vi "ExampleGreyscaleImageData.vi"(8 "error in (no error)":errorcluster, 11 "Image Size":T3={"Width"=3, "Height"=2}) -> (0 "error out":errorcluster, 3 "Greyscale Destination Image":T1, 5 "Greyscale Data":u8[][](array[numeric]), 7 "Greyscale Pixmap Data":T2)   [LabVIEW 2020, in "test.lvlib" / "01_Image.lvclass"]
uses:
  01_Image.lvclass
  common/Image Size (Integer).ctl
  <vilib>/picture/picture.llb/imagedata.ctl
  image/Greyscale Image.ctl
  image/New Image (Greyscale Preallocated).vi
  image/Copy Array to Image (Greyscale).vi
  image/New Image (Greyscale Preallocated).vi/6598b9e0-8a08-46f5-91fd-ca1b87217137.vi
  <vilib>/Utility/error.llb/Error Cluster From Error Code.vi
  01_Image.lvclass/01_Image.ctl
  image/image.lvlib
  common/common.lvlib
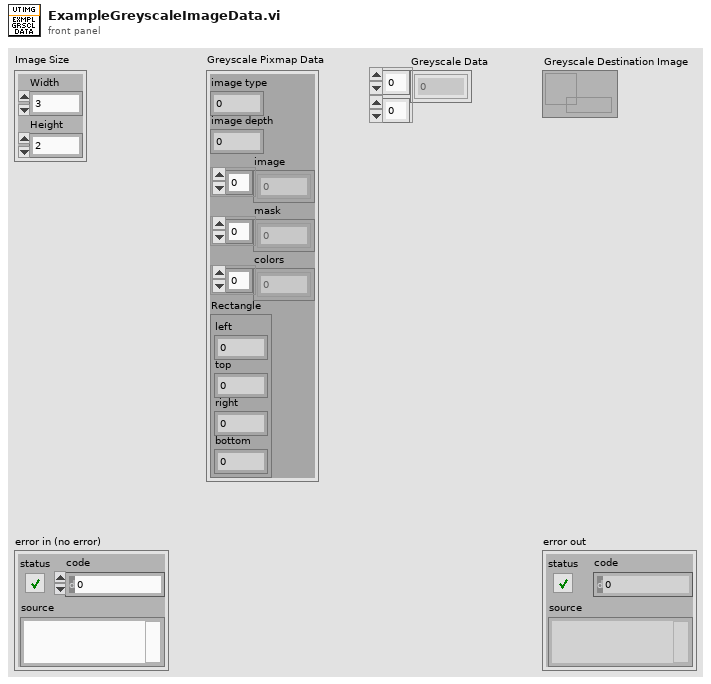
[diagram p1: front panel]
types:
  T1 = typedef "image.lvlib/Greyscale Image.ctl" = refnum<data-value>
  T2 = typedef "imagedata.ctl" = cluster{"image type":i32, "image depth":i32, "image":u8[], "mask":u8[], "colors":u32[], "Rectangle":cluster{"left":i16, "top":i16, "right":i16, "bottom":i16}}
  T3 = typedef "common.lvlib/Image Size (Integer).ctl" = cluster{"Width":u16, "Height":u16}
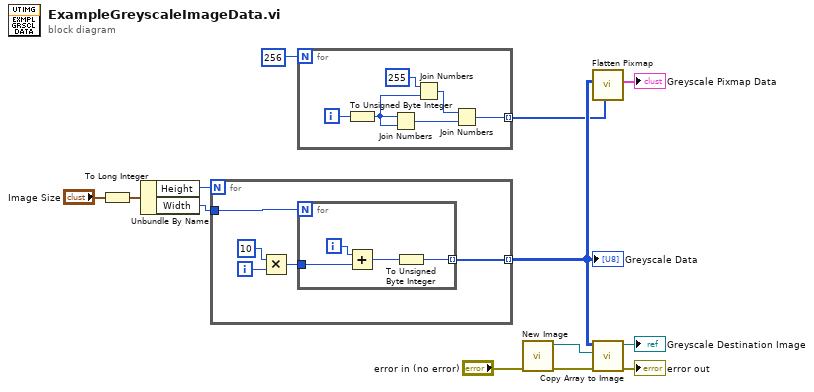
[diagram p0: block diagram]
diagram:
  n1 = To Long Integer(number="Image Size") -> (32bit integer=w12:cluster{"Width":i32, "Height":i32})
  n2 = Unbundle By Name(w12) -> ("Height"=w6:i32, "Width"=w5:i32)
  n3 = for {
    N: w6 -> [_]
    tunnel: w5 -> [w18]
    tunnel: [w14] -> w4 mode=indexing
    i -> [w17]
    n4 = Multiply(x=10, y=w17) -> (x*y=w15:i32)
    n5 = for {
      N: w18 -> [_]
      tunnel: w15 -> [w22]
      tunnel: [w19] -> w14 mode=indexing
      i -> [w21]
      n6 = Add(x=w21, y=w22) -> (x+y=w20:i32)
      n7 = To Unsigned Byte Integer(number=w20) -> (unsigned 8bit integer=w19:u8)
    }
  }
  "Greyscale Data" <- w4
  n8 = for {
    N: 256 -> [_]
    tunnel: [w23] -> w1 mode=indexing
    i -> [w28]
    n9 = To Unsigned Byte Integer(number=w28) -> (unsigned 8bit integer=w26:u8)
    n10 = Join Numbers(hi=w26, lo=w26) -> ((hi.lo)=w25:u16)
    n11 = Join Numbers(hi=u8 255, lo=w26) -> ((hi.lo)=w24:u16)
    n12 = Join Numbers(hi=w24, lo=w25) -> ((hi.lo)=w23:u32)
  }
  n13 = call-poly "New Image.vi"("error in (no error)"="error in (no error)") -> ("error out"=w9:errorcluster, "New Greyscale Image"=w7:T1)  [unwired: 9 in]
  n14 = call <vilib>:"Flatten Pixmap.vi"("colors"=w1, "8-bit pixmap"=w4) -> ("image data"=→"Greyscale Pixmap Data":T2)  [unwired: 9 in]
  n15 = call-poly "Copy Array to Image.vi"("error in (no error)"=w9, "Greyscale Destination Image"=w7, "U8 Greyscale Data"=w4) -> ("error out"=→"error out":errorcluster, "Greyscale Destination Image (duplicate)"=→"Greyscale Destination Image":T1)  [unwired: 7 in]
